vi "Read Measurement (Noise).vi"(0 "VISA resource name":refnum<visa-resource-name>, 1 "Measure Type (0: Zero)":i32(ring) items=["Zero", "One", "Both"], 5 "Source (0: Channel 1)":i32(ring) items=["Channel 1", "Channel 2", "Channel 3", "Channel 4", "Function 1", "Function 2", "Function 3", "Function 4", "Memory 1", "Memory 2", "Memory 3", "Memory 4", "Equalized"], 7 "Units (0: Volt)":i32(ring) items=["Volt", "UNIT"], 9 "Maximum Time (10000ms)":u32=10000, 11 "error in (no error)":errorcluster) -> (4 "VISA resource name out":refnum<visa-resource-name>, 10 "Noise Value":dbl, 15 "error out":errorcluster)   [LabVIEW 2013, in "Agilent 90000 Series.lvlib"]
doc: "Returns the result of a noise measurement.\n\nThis VI initiates an acquisition on the channel that the end-user defines. It then waits for the acquisition to complete, obtains a waveform measurement on the channel the end-user specifies, and returns the measurement value."
uses:
  Agilent 90000 Series.lvlib
  Low Level/Fetch Measurement (Noise).vi
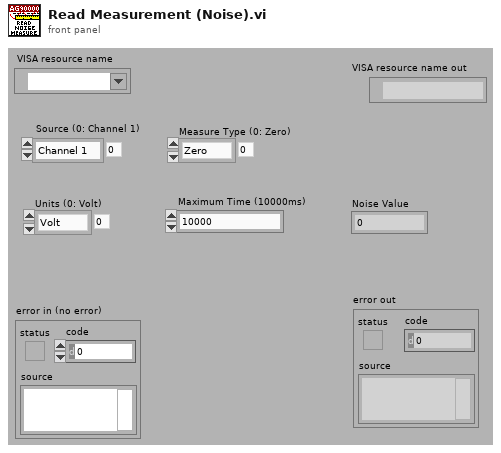
[diagram p1: front panel]
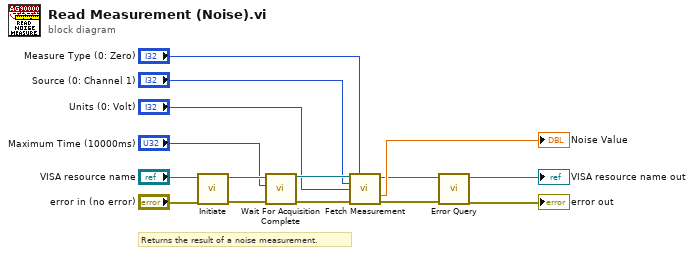
[diagram p0: block diagram]
diagram:
  # "Returns the result of a noise measurement."
  n1 = call "Initiate.vi"("error in (no error)"="error in (no error)", "VISA resource name"="VISA resource name") -> ("error out"=w10:errorcluster, "VISA resource name out"=w13:refnum<visa-resource-name>)  [unwired: 8 out]
  n2 = call "Wait For Acquisition Complete.vi"("error in (no error)"=w10, "Maximum Time (10000ms)"="Maximum Time (10000ms)", "VISA resource name"=w13) -> ("error out"=w5:errorcluster, "VISA resource name out"=w6:refnum<visa-resource-name>)  [unwired: 7 out]
  n3 = call-poly "Fetch Measurement.vi"("VISA resource name"=w6, "Measure Type (0: Zero)"="Measure Type (0: Zero)", "Source (0: Channel 1)"="Source (0: Channel 1)", "Units (0: Volt)"="Units (0: Volt)", "error in (no error)"=w5) -> ("VISA resource name out"=w4:refnum<visa-resource-name>, "Noise Value"=→"Noise Value":dbl, "error out"=w3:errorcluster)  [unwired: 1 in, 7 out]
  n4 = call "Error Query.vi"("error in (no error)"=w3, "VISA resource name"=w4) -> ("error out"=→"error out":errorcluster, "VISA resource name out"=→"VISA resource name out":refnum<visa-resource-name>)  [unwired: 8 out]
